vi "Get U max Haskel.vi"(11 "Stand in":refnum<class "Stand.lvclass">) -> (3 "U max [V]":dbl)   [LabVIEW 2019, in "Stand.lvclass"]
uses:
  Stand.lvclass
  Stand.lvclass/Stand.ctl
  FPGA/TypeDef/AI index.ctl
  AI_class/AI.lvclass/AI.ctl
  AnalogComparator_class/AnalogComparator.lvclass/AnalogComparator.ctl
  AnalogComparator_class/GetStatus.vi
  Global/Global Constant.vi
  AI_class/AI.lvclass
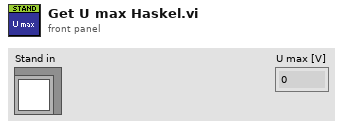
[diagram p1: front panel]
types:
  T1 = typedef "AI index.ctl" = u8
  T2 = typedef "AI_Data.ctl" = cluster{"Stat Data":T3, "OutOfRangeMax":bool, "OutOfRangeMin":bool, "HIHI":bool, "HI":bool, "LO":bool, "LOLO":bool}
  T3 = typedef "AI Statistics Data.ctl" = cluster{"raw mean":dbl, "scl mean":dbl, "raw mean 1Hz":dbl, "scl mean 1Hz":dbl}
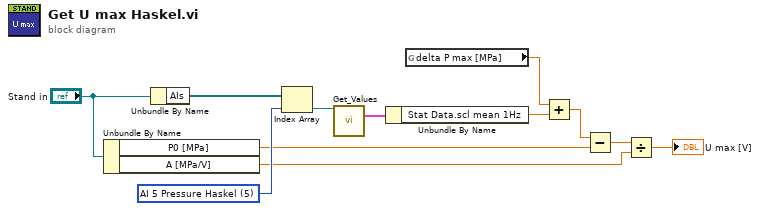
[diagram p0: block diagram]
diagram:
  w11 = T1 5 items=["AI 0 Cooling Station Level", "AI 1 Cooling Station Temp", "AI 2 Oil Supply Level", "AI 3 Oil Supply Temp", "AI 4 ", "AI 5 Pressure Haskel", "AI 6 Pressure DUT", "AI 7 Pressure Chamber", "AI 8 Pressure Air inlet", "AI 9 Pressure Air outlet", "AI 10 Pressure Messure Line", "AI 11 DUT 2", "AI 12 Chamber 2"] ("AI index")
  n1 = Unbundle By Name("Stand in") -> ("P0 [MPa]"=w2:dbl, "A [MPa/V]"=w7:dbl)
  n2 = Unbundle By Name("Stand in") -> ("AIs"=w12:refnum<class "AI.lvclass">[])
  n3 = Index Array(array=w12, index=w11) -> (element=w10:refnum<class "AI.lvclass">)
  n4 = call "Get_Values.vi"("reference in"=w10) -> ("Data"=w9:T2)  [unwired: 14 in]
  n5 = Unbundle By Name(w9) -> ("Stat Data.scl mean 1Hz"=w4:dbl)
  n6 = global read "Global Constant.vi" "delta P max [MPa]"() -> (w5:dbl)
  n7 = Add(x=w5, y=w4) -> (x+y=w3:dbl)
  n8 = Subtract(x=w3, y=w2) -> (x-y=w1:dbl)
  n9 = Divide(x=w1, y=w7) -> (x/y=→"U max [V]":dbl)
